vi "Readout File Props.vi"(8 "error in (no error)":errorcluster, 9 "filename without extension":string, 10 "extension":string, 11 "file path":path) -> (0 "error out":errorcluster, 3 "Exec":T1)   [LabVIEW 2022 SP3]
uses:
  TDs/FileProps.ctl
  3341bc90-c10b-4d5e-840b-d54f322447ca.vi
panel:
  in  "Load":bool
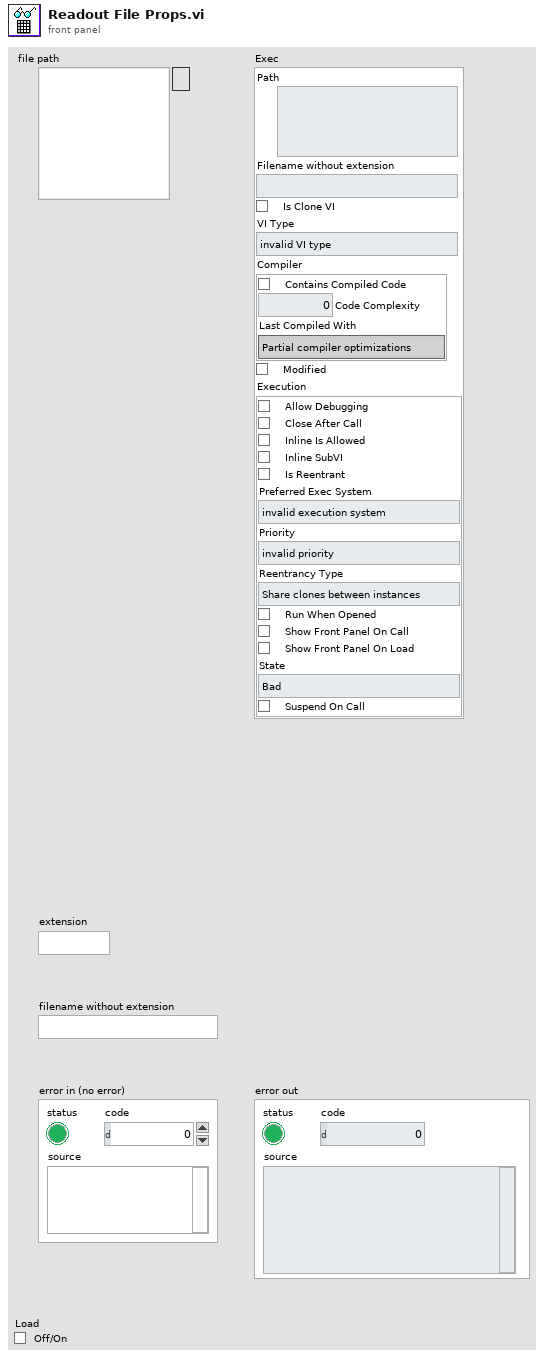
[diagram p1: front panel]
types:
  T1 = typedef "FileProps.ctl" = cluster{"Path":path, "Filename without extension":string, "Is Clone VI":bool, "VI Type":enum32{"invalid VI type", "Standard VI", "Control VI", "Global VI", "Polymorphic VI", "Configuration VI", "SubSystem", "Facade VI", "Method VI", "Statechart Diagram VI"}, "Compiler":cluster{"Contains Compiled Code":bool, "Code Complexity":sgl, "Last Compiled With":enum16{"Partial compiler optimizations", "Full compiler optimizations"}}, "Modified":bool, "Execution":cluster{"Allow Debugging":bool, "Close After Call":bool, "Inline Is Allowed":bool, "Inline SubVI":bool, "Is Reentrant":bool, "Preferred Exec System":enum32{"invalid execution system", "user interface", "standard", "instrument i/o", "data acquisition", "other 1", "other 2", "same as caller"}, "Priority":enum32{"invalid priority", "background priority", "normal priority", "above normal priority", "high priority", "time critical priority", "subroutine"}, "Reentrancy Type":enum16{"Share clones between instances", "Preallocate clone for each instance"}, "Run When Opened":bool, "Show Front Panel On Call":bool, "Show Front Panel On Load":bool, "State":enum32{"Bad", "Idle", "Run top level", "Running"}, "Suspend On Call":bool}}
  T2 = enum32{"Invalid", "Standard", "Closed", "Hidden", "Minimized", "Maximized"}
  T3 = enum32{"invalid execution system", "user interface", "standard", "instrument i/o", "data acquisition", "other 1", "other 2", "same as caller"}
  T4 = enum32{"invalid priority", "background priority", "normal priority", "above normal priority", "high priority", "time critical priority", "subroutine"}
  T5 = enum16{"Share clones between instances", "Preallocate clone for each instance"}
  T6 = enum32{"Bad", "Idle", "Run top level", "Running"}
  T7 = enum32{"invalid VI type", "Standard VI", "Control VI", "Global VI", "Polymorphic VI", "Configuration VI", "SubSystem", "Facade VI", "Method VI", "Statechart Diagram VI"}
  T8 = typedef "LVLastCompiledWithTypeDef.ctl" = enum16{"Partial compiler optimizations", "Full compiler optimizations"}
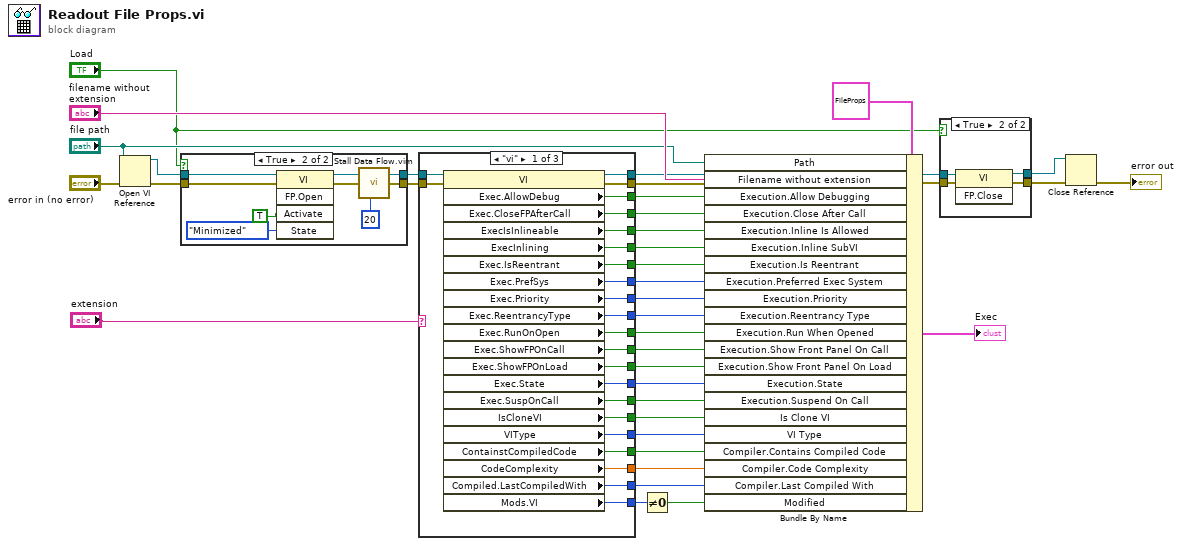
[diagram p0: block diagram]
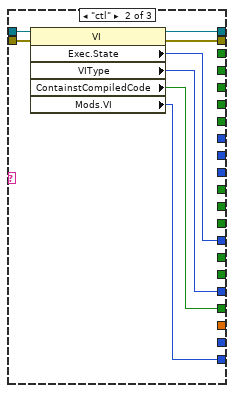
[diagram p2: hidden frame]
diagram:
  n1 = Open VI Reference(vi path="file path", error in (no error)="error in (no error)") -> (vi reference=w15:refnum<vi>, error out=w14:errorcluster)  [unwired: 4 in]
  n2 = case shown="True" "Load" {
    tunnel: w15 -> [w38 w42]
    tunnel: w14 -> [w37 w41]
    tunnel: [w37 w40] -> w13
    tunnel: [w38 w39] -> w12
    frame False {
    }
    frame True {
      n3 = invoke class="VI" method="FP.Open"(reference=w42, error in=w41, "Activate"=TRUE ("Activate?"), "State"=T2."Minimized") -> (reference out=w39:refnum<vi>, error out=w46:errorcluster)  [unwired: 1 in, 3 out]
      n4 = call "Stall Data Flow.vim"("value in"=w46, "milliseconds to wait"=u32 20) -> ("value out"=w40:errorcluster)  [unwired: 1 out]
    }
  }
  n5 = case shown="\"vi\"" "extension" {
    tunnel: [w69 w77 _] -> w36
    tunnel: [w68 _ _] -> w35
    tunnel: [w67 _ _] -> w34
    tunnel: [w66 _ _] -> w33
    tunnel: [w65 _ _] -> w32
    tunnel: [w64 _ _] -> w31
    tunnel: [w63 _ _] -> w30
    tunnel: [w62 _ _] -> w29
    tunnel: [w61 _ _] -> w28
    tunnel: [w60 _ _] -> w27
    tunnel: [w59 _ _] -> w26
    tunnel: [w58 _ _] -> w25
    tunnel: [w57 w76 _] -> w24
    tunnel: [w56 _ _] -> w23
    tunnel: [w55 _ _] -> w21
    tunnel: w13 -> [w54 w75 w78]
    tunnel: w12 -> [w53 w74 w79]
    tunnel: [w52 w73 w79] -> w11
    tunnel: [w51 w72 w78] -> w10
    tunnel: [w50 w71 _] -> w6
    tunnel: [w49 _ _] -> w5
    tunnel: [w48 _ _] -> w4
    tunnel: [w47 w70 _] -> w2
    frame "vi" {
      n6 = property class="VI"(reference=w53, error in=w54) -> (reference out=w52:refnum<vi>, error out=w51:errorcluster, "Exec.AllowDebug"=w55:bool, "Exec.CloseFPAfterCall"=w67:bool, "ExecIsInlineable"=w66:bool, "ExecInlining"=w65:bool, "Exec.IsReentrant"=w64:bool, "Exec.PrefSys"=w63:T3, "Exec.Priority"=w62:T4, "Exec.ReentrancyType"=w61:T5, "Exec.RunOnOpen"=w60:bool, "Exec.ShowFPOnCall"=w59:bool, "Exec.ShowFPOnLoad"=w58:bool, "Exec.State"=w57:T6, "Exec.SuspOnCall"=w56:bool, "IsCloneVI"=w68:bool, "VIType"=w69:T7, "ContainstCompiledCode"=w50:bool, "CodeComplexity"=w49:sgl, "Compiled.LastCompiledWith"=w48:T8, "Mods.VI"=w47:u64)
    }
    frame "ctl" {
      n7 = property class="VI"(reference=w74, error in=w75) -> (reference out=w73:refnum<vi>, error out=w72:errorcluster, "Exec.State"=w76:T6, "VIType"=w77:T7, "ContainstCompiledCode"=w71:bool, "Mods.VI"=w70:u64)
    }
    frame Default {
    }
  }
  n8 = Not Equal To 0?(x=w2) -> (x != 0?=w1:bool)
  n9 = Bundle By Name(cluster=T1 {"Path"=path "", "Filename without extension"="", "Is Clone VI"=FALSE, "VI Type"=enum."invalid VI type", "Compiler"={"Contains Compiled Code"=FALSE, "Code Complexity"=0.0, "Last Compiled With"=enum."Partial compiler optimizations"}, "Modified"=FALSE, "Execution"={"Allow Debugging"=FALSE, "Close After Call"=FALSE, "Inline Is Allowed"=FALSE, "Inline SubVI"=FALSE, "Is Reentrant"=FALSE, "Preferred Exec System"=enum."invalid execution system", "Priority"=enum."invalid priority", "Reentrancy Type"=enum."Share clones between instances", "Run When Opened"=FALSE, "Show Front Panel On Call"=FALSE, "Show Front Panel On Load"=FALSE, "State"=enum."Bad", "Suspend On Call"=FALSE}}, "Path"="file path", "Filename without extension"="filename without extension", "Execution.Allow Debugging"=w21, "Execution.Close After Call"=w34, "Execution.Inline Is Allowed"=w33, "Execution.Inline SubVI"=w32, "Execution.Is Reentrant"=w31, "Execution.Preferred Exec System"=w30, "Execution.Priority"=w29, "Execution.Reentrancy Type"=w28, "Execution.Run When Opened"=w27, "Execution.Show Front Panel On Call"=w26, "Execution.Show Front Panel On Load"=w25, "Execution.State"=w24, "Execution.Suspend On Call"=w23, "Is Clone VI"=w35, "VI Type"=w36, "Compiler.Contains Compiled Code"=w6, "Compiler.Code Complexity"=w5, "Compiler.Last Compiled With"=w4, "Modified"=w1) -> (→"Exec":T1)
  n10 = case shown="True" "Load" {
    tunnel: w11 -> [w81 w85]
    tunnel: w10 -> [w80 w84]
    tunnel: [w80 w83] -> w9
    tunnel: [w81 w82] -> w8
    frame False {
    }
    frame True {
      n11 = invoke class="VI" method="FP.Close"(reference=w85, error in=w84) -> (reference out=w82:refnum<vi>, error out=w83:errorcluster)  [unwired: 1 in, 1 out]
    }
  }
  n12 = Close Reference(reference=w8, error in (no error)=w9) -> (error out=→"error out":errorcluster)
